vi "PickAndPlace.vi"(0 "Operations":T1={"GoToToolPos"=TRUE, "PickTool"=TRUE, "GoToSenPCB"=TRUE, "PickSiPCB"=TRUE, "GoToBP"=TRUE, "DropTool"=TRUE}, 1 "VacuumStates":path=path "C:/Users/TTUHEP/Documents/LabVIEW/GantryPrograms/Configs/PickPlaceVacuumStates.json", 2 "AssemblyPositions":path=path "C:/Users/TTUHEP/Documents/LabVIEW/GantryPrograms/Configs/BaseplatePositions.txt", 5 "AssmbType":enum16{"Sensor", "PCB"}(ring)=enum."PCB", 7 "Zone":enum16{"ZoneA", "ZoneB", "ZoneC", "ZoneD"}(ring), 9 "Position":enum16{"1", "2"}(ring), 11 "Error In":errorcluster, 12 "PUT_Positions":path=path "C:/Users/TTUHEP/Documents/LabVIEW/GantryPrograms/Configs/PUT_Positions.txt", 13 "SiPositions":path=path "C:/Users/TTUHEP/Documents/LabVIEW/GantryPrograms/Configs/SensorPositions.txt", 14 "PCBPositions":path=path "C:/Users/TTUHEP/Documents/LabVIEW/GantryPrograms/Configs/PCBPositions.txt") -> (4 "Log":string, 15 "Error Out":errorcluster)   [LabVIEW 2019]
panel:
  out "Assembly_XYZU":dbl[](array[numeric])
  out "PUT_XYZU":dbl[](array[numeric])
  out "PUT rotation":dbl
  in  "FastZDrop":dbl=65.0
  in  "FastZToolPick":dbl=85.0
  in  "FastZSiPCBPick":dbl=65.0
  in  "LineNo":u8
  in  "ZSpeed":dbl=10.0
  in  "XYSpeed":dbl=100.0
  out "SiPCBXYZU":dbl[](array[numeric])
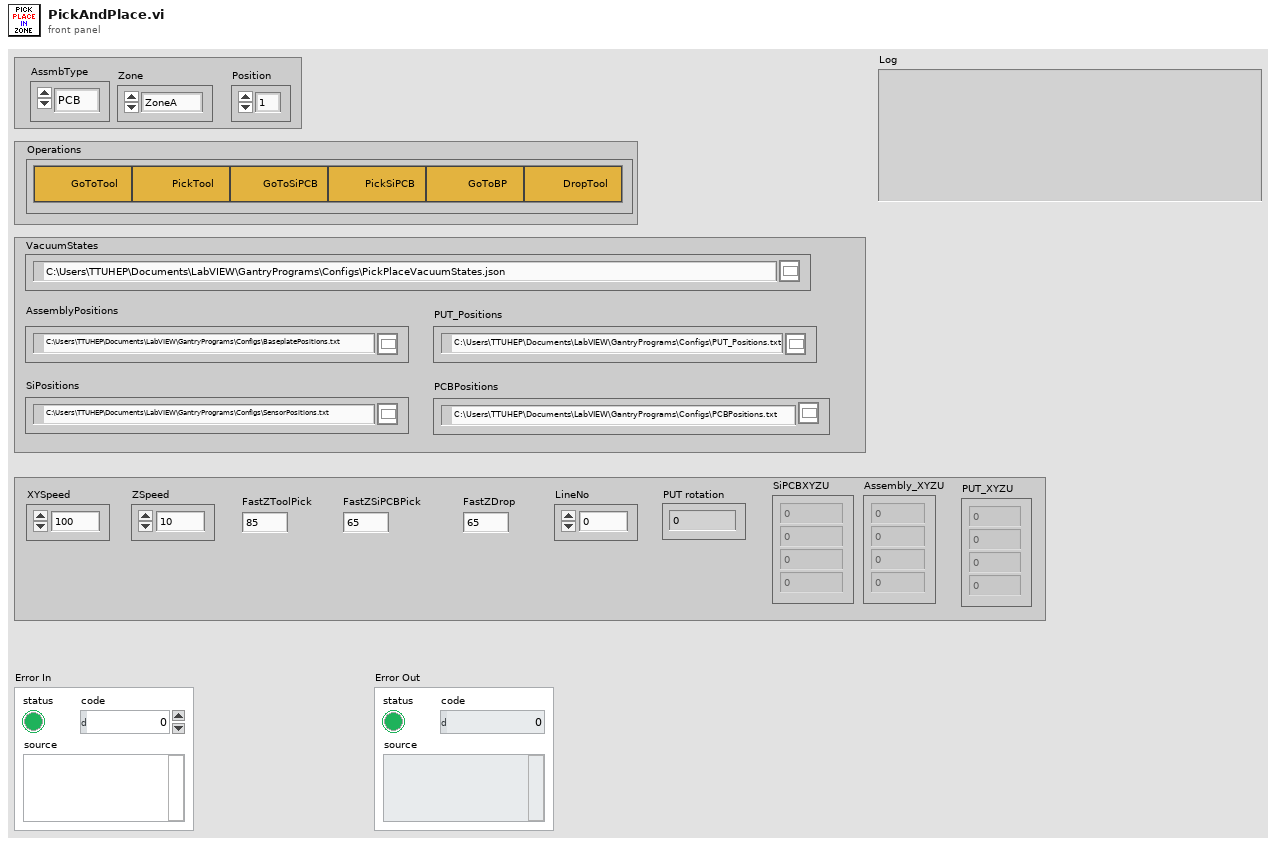
[diagram p1: front panel]
types:
  T1 = cluster{"GoToToolPos":bool, "PickTool":bool, "GoToSenPCB":bool, "PickSiPCB":bool, "GoToBP":bool, "DropTool":bool}
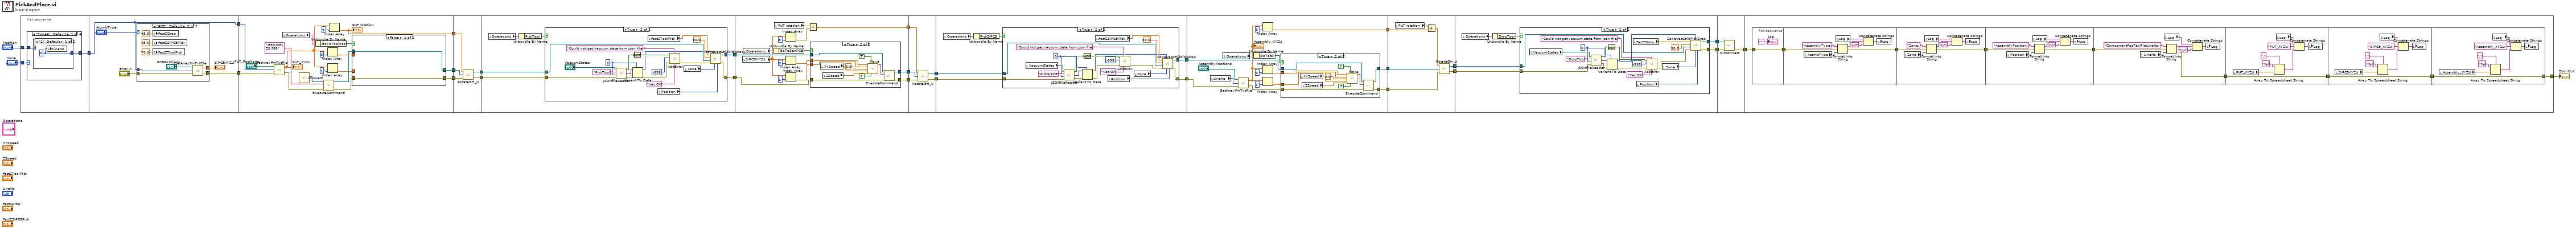
[diagram p0: block diagram]
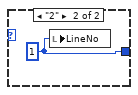
[diagram p2: hidden frame]
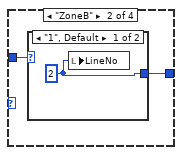
[diagram p3: hidden frame]
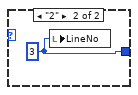
[diagram p4: hidden frame]
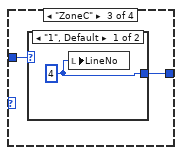
[diagram p5: hidden frame]
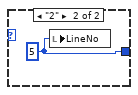
[diagram p6: hidden frame]
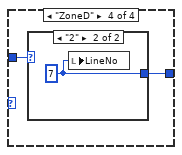
[diagram p7: hidden frame]
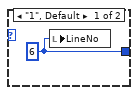
[diagram p8: hidden frame]
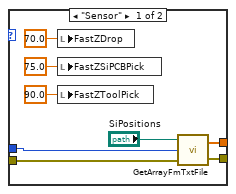
[diagram p9: hidden frame]
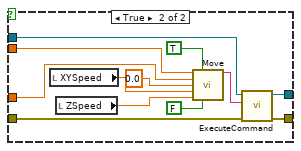
[diagram p10: hidden frame]
diagram:
  n1 = flat-sequence {
    tunnel: [w29] -> w8
    tunnel: "Zone" -> [w31]
    tunnel: "Position" -> [w30]
    tunnel: [w50] -> w9
    tunnel: w8 -> [w48]
    tunnel: [w48] -> w6
    tunnel: [w77] -> w28
    tunnel: [w76] -> w27
    tunnel: [w75] -> w26
    tunnel: w9 -> [w71]
    tunnel: w6 -> [w74]
    tunnel: w28 -> [w106]
    tunnel: w27 -> [w105]
    tunnel: w26 -> [w104]
    tunnel: [w103] -> w25
    tunnel: [w102] -> w24
    tunnel: w25 -> [w110]
    tunnel: w24 -> [w109]
    tunnel: [w108] -> w23
    tunnel: [w107] -> w22
    tunnel: w23 -> [w143]
    tunnel: w22 -> [w142]
    tunnel: [w136] -> w21
    tunnel: [w141] -> w20
    tunnel: [w140] -> w19
    tunnel: w21 -> [w169]
    tunnel: w20 -> [w168]
    tunnel: w19 -> [w167]
    tunnel: [w166] -> w18
    tunnel: [w165] -> w17
    tunnel: w18 -> [w173]
    tunnel: w17 -> [w172]
    tunnel: [w171] -> w16
    tunnel: [w170] -> w15
    tunnel: w16 -> [w205]
    tunnel: w15 -> [w204]
    tunnel: [w202] -> w14
    tunnel: [w201] -> w13
    tunnel: [w200] -> w12
    tunnel: w14 -> [w235]
    tunnel: w13 -> [w234]
    tunnel: w12 -> [w232]
    tunnel: [w230] -> w11
    tunnel: [w229] -> w10
    tunnel: w11 -> [w239]
    tunnel: w10 -> [w238]
    tunnel: [w237] -> w4
    tunnel: [w236] -> w3
    tunnel: w4 -> [w267]
    tunnel: w3 -> [w266]
    tunnel: [w265] -> w1
    tunnel: [w270] -> w2
    tunnel: w1 -> [w268]
    frame #0 {
      n2 = case shown="\"ZoneA\", Default" w31 {
        tunnel: w30 -> [w33 w37 w41 w45]
        tunnel: [w32 w36 w40 w44] -> w29
        frame "ZoneA", Default {
          n3 = case shown="\"1\", Default" w33 {
            tunnel: [w34 w35] -> w32
            frame "1", Default {
              w34 = u8 0 ("LineNo")
              n4 = local write "LineNo"(w34) -> ()
            }
            frame "2" {
              w35 = u8 1 ("LineNo")
              n5 = local write "LineNo"(w35) -> ()
            }
          }
        }
        frame "ZoneB" {
          n6 = case shown="\"1\", Default" w37 {
            tunnel: [w38 w39] -> w36
            frame "1", Default {
              w38 = u8 2 ("LineNo")
              n7 = local write "LineNo"(w38) -> ()
            }
            frame "2" {
              w39 = u8 3 ("LineNo")
              n8 = local write "LineNo"(w39) -> ()
            }
          }
        }
        frame "ZoneC" {
          n9 = case shown="\"1\", Default" w41 {
            tunnel: [w42 w43] -> w40
            frame "1", Default {
              w42 = u8 4 ("LineNo")
              n10 = local write "LineNo"(w42) -> ()
            }
            frame "2" {
              w43 = u8 5 ("LineNo")
              n11 = local write "LineNo"(w43) -> ()
            }
          }
        }
        frame "ZoneD" {
          n12 = case shown="\"2\"" w45 {
            tunnel: [w46 w47] -> w44
            frame "1", Default {
              w46 = u8 6 ("LineNo")
              n13 = local write "LineNo"(w46) -> ()
            }
            frame "2" {
              w47 = u8 7 ("LineNo")
              n14 = local write "LineNo"(w47) -> ()
            }
          }
        }
      }
    }
    frame #1 {
      n15 = case shown="\"PCB\", Default" "AssmbType" {
        tunnel: w48 -> [w59 w67]
        tunnel: [w58 w66] -> w52
        tunnel: "Error In" -> [w57 w65]
        tunnel: [w56 w64] -> w50
        frame "Sensor" {
          n16 = local write "FastZDrop"(70.0 ("FastZDrop")) -> ()
          n17 = local write "FastZSiPCBPick"(75.0 ("FastZSiPCBPick")) -> ()
          n18 = local write "FastZToolPick"(90.0 ("FastZToolPick")) -> ()
          n19 = call "GetArrayFmTxtFile.vi"("error in"=w57, "LineNo."=w59, "TextFile"="SiPositions") -> ("error out"=w56:errorcluster, "Array"=w58:dbl[])
        }
        frame "PCB", Default {
          n20 = local write "FastZDrop"(45.0 ("FastZDrop")) -> ()
          n21 = local write "FastZSiPCBPick"(45.0 ("FastZSiPCBPick")) -> ()
          n22 = local write "FastZToolPick"(70.0 ("FastZToolPick")) -> ()
          n23 = call "GetArrayFmTxtFile.vi"("error in"=w65, "LineNo."=w67, "TextFile"="PCBPositions") -> ("error out"=w64:errorcluster, "Array"=w66:dbl[])
        }
      }
      "SiPCBXYZU" <- w52
    }
    frame #2 {
      n24 = call "GetArrayFmTxtFile.vi"("error in"=w71, "LineNo."=w74, "TextFile"="PUT_Positions") -> ("error out"=w72:errorcluster, "Array"=w69:dbl[])
      "PUT_XYZU" <- w69
      n25 = local read "Operations"() -> (w84:T1)
      n26 = call "Connect.vi"() -> ("controller"=w70:refnum<k24>)  [unwired: 10 in, 1 out]
      n27 = Unbundle By Name(w84) -> ("GoToToolPos"=w83:bool)
      n28 = call "ExecuteCommand.vi"("error in (no error)"=w72, "Command Code"="G90\nG1 Z0 F50", "controller in"=w70) -> ("error out"=w87:errorcluster, "controller out"=w86:refnum<k24>)  [unwired: 6 in, 1 out]
      n29 = Index Array(array=w69, index=0) -> (element=w79:dbl)
      n30 = Index Array(array=w69, index=1) -> (element=w78:dbl)
      n31 = Index Array(array=w69, index=3) -> (element=w75:dbl)
      "PUT rotation" <- w75
      n32 = case shown="False" w83 {
        tunnel: w86 -> [w89 w98]
        tunnel: w87 -> [w88 w97]
        tunnel: [w88 w96] -> w77
        tunnel: [w89 w95] -> w76
        tunnel: w79 -> [_ w94]
        tunnel: w78 -> [_ w93]
        frame False {
        }
        frame True {
          n33 = local read "XYSpeed"() -> (w91:dbl)
          n34 = local read "ZSpeed"() -> (w90:dbl)
          n35 = call "Move.vi"("X"=w94, "Absolute"=TRUE, "Y"=w93, "Z"=0.0, "SpeedXY (mm/s)"=w91, "SpeedZ (mm/s)"=w90, "Move Z first"=FALSE) -> ("Position Gcode"=w99:string)  [unwired: 8 in]
          n36 = call "ExecuteCommand.vi"("error in (no error)"=w97, "Command Code"=w99, "controller in"=w98) -> ("error out"=w96:errorcluster, "controller out"=w95:refnum<k24>)  [unwired: 6 in, 1 out]
        }
      }
    }
    frame #3 {
      n37 = call "RotateGH_U.vi"("error in (no error)"=w106, "controller in"=w105, "U"=w104) -> ("error out"=w103:errorcluster, "controller out"=w102:refnum<k24>)
    }
    frame #4 {
      n38 = local read "Operations"() -> (w112:T1)
      n39 = Unbundle By Name(w112) -> ("PickTool"=w111:bool)
      n40 = case shown="True" w111 {
        tunnel: w110 -> [w114 w121]
        tunnel: w109 -> [w113 w134]
        tunnel: [w114 w117] -> w108
        tunnel: [w113 w116] -> w107
        frame False {
        }
        frame True {
          w124 = u8 0
          n41 = call "JSONfileReader.vi"("error in"=w121, "Variant"=w124, "ItemName"="PickTool", "FileIn"="VacuumStates") -> ("error out"=w119:errorcluster, "Data"=w123:variant, "Found"=w128:bool)
          n42 = Not(x=w128) -> (.not. x?=w129:bool)
          n43 = Variant To Data(error in=w119, type=w124, Variant=w123) -> (data=w122:u8, error out=w118:errorcluster)
          n44 = local read "FastZToolPick"() -> (w115:dbl)
          n45 = local read "Position"() -> (w133:enum16{"1", "2"})
          n46 = call "AddError.vi"("NoErrorMessage"="Vac OK", "ErrorMessage"="Could not get vacuum state from json file.", "error in"=w118, "code"=-998, "Error?"=w129) -> ("Error out"=w120:errorcluster)  [unwired: 6 in]
          n47 = local read "Zone"() -> (w132:enum16{"ZoneA", "ZoneB", "ZoneC", "ZoneD"})
          n48 = call "ZoneVacCtrldPickDrop.vi"("Position"=w133, "Zone"=w132, "VacuumState"=w122, "error in (no error)"=w120, "controller in"=w134, "Zspeed"=50.0, "Z"=w115) -> ("error out"=w117:errorcluster, "controller out"=w116:refnum<k24>)  [unwired: 3 in]
        }
      }
    }
    frame #5 {
      n49 = local read "SiPCBXYZU"() -> (w139:dbl[])
      n50 = local read "Operations"() -> (w147:T1)
      n51 = Unbundle By Name(w147) -> ("GoToSenPCB"=w148:bool)
      n52 = local read "PUT rotation"() -> (w138:dbl)
      n53 = Index Array(array=w139, index=3) -> (element=w137:dbl)
      n54 = Index Array(array=w139, index=0) -> (element=w149:dbl)
      n55 = Index Array(array=w139, index=1) -> (element=w150:dbl)
      n56 = Add(x=w138, y=w137) -> (x+y=w136:dbl)
      n57 = case shown="True" w148 {
        tunnel: w142 -> [w152 w161]
        tunnel: w143 -> [w151 w160]
        tunnel: [w151 w159] -> w140
        tunnel: [w152 w158] -> w141
        tunnel: w149 -> [_ w157]
        tunnel: w150 -> [_ w156]
        frame False {
        }
        frame True {
          n58 = local read "XYSpeed"() -> (w153:dbl)
          n59 = local read "ZSpeed"() -> (w154:dbl)
          n60 = call "Move.vi"("X"=w157, "Absolute"=TRUE, "Y"=w156, "Z"=0.0, "SpeedXY (mm/s)"=w153, "SpeedZ (mm/s)"=w154, "Move Z first"=FALSE) -> ("Position Gcode"=w162:string)  [unwired: 8 in]
          n61 = call "ExecuteCommand.vi"("error in (no error)"=w160, "Command Code"=w162, "controller in"=w161) -> ("error out"=w159:errorcluster, "controller out"=w158:refnum<k24>)  [unwired: 6 in, 1 out]
        }
      }
    }
    frame #6 {
      n62 = call "RotateGH_U.vi"("error in (no error)"=w167, "controller in"=w168, "U"=w169) -> ("error out"=w165:errorcluster, "controller out"=w166:refnum<k24>)
    }
    frame #7 {
      n63 = local read "Operations"() -> (w174:T1)
      n64 = Unbundle By Name(w174) -> ("PickSiPCB"=w175:bool)
      n65 = case shown="True" w175 {
        tunnel: w172 -> [w177 w186]
        tunnel: w173 -> [w176 w178]
        tunnel: [w177 w182] -> w170
        tunnel: [w176 w181] -> w171
        frame False {
        }
        frame True {
          w189 = u8 0
          n66 = local read "VacuumStates"() -> (w180:path)
          n67 = call "JSONfileReader.vi"("error in"=w186, "Variant"=w189, "ItemName"="PickSiPCB", "FileIn"=w180) -> ("error out"=w184:errorcluster, "Data"=w188:variant, "Found"=w193:bool)
          n68 = Not(x=w193) -> (.not. x?=w194:bool)
          n69 = Variant To Data(error in=w184, type=w189, Variant=w188) -> (data=w187:u8, error out=w183:errorcluster)
          n70 = local read "FastZSiPCBPick"() -> (w179:dbl)
          n71 = local read "Position"() -> (w197:enum16{"1", "2"})
          n72 = call "AddError.vi"("NoErrorMessage"="Vac OK", "ErrorMessage"="Could not get vacuum state from json file.", "error in"=w183, "code"=-998, "Error?"=w194) -> ("Error out"=w185:errorcluster)  [unwired: 6 in]
          n73 = local read "Zone"() -> (w196:enum16{"ZoneA", "ZoneB", "ZoneC", "ZoneD"})
          n74 = call "ZoneVacCtrldPickDrop.vi"("Position"=w197, "Zone"=w196, "VacuumState"=w187, "error in (no error)"=w185, "controller in"=w178, "Zspeed"=50.0, "Z"=w179) -> ("error out"=w182:errorcluster, "controller out"=w181:refnum<k24>)  [unwired: 3 in]
        }
      }
    }
    frame #8 {
      n75 = local read "LineNo"() -> (w206:u8)
      n76 = local read "Operations"() -> (w214:T1)
      n77 = call "GetArrayFmTxtFile.vi"("error in"=w204, "LineNo."=w206, "TextFile"="AssemblyPositions") -> ("error out"=w203:errorcluster, "Array"=w199:dbl[])
      "Assembly_XYZU" <- w199
      n78 = Unbundle By Name(w214) -> ("GoToBP"=w213:bool)
      n79 = Index Array(array=w199, index=3) -> (element=w200:dbl)
      n80 = Index Array(array=w199, index=0) -> (element=w212:dbl)
      n81 = Index Array(array=w199, index=1) -> (element=w211:dbl)
      n82 = case shown="True" w213 {
        tunnel: w205 -> [w216 w225]
        tunnel: w203 -> [w215 w224]
        tunnel: [w215 w223] -> w202
        tunnel: [w216 w222] -> w201
        tunnel: w212 -> [_ w221]
        tunnel: w211 -> [_ w220]
        frame False {
        }
        frame True {
          n83 = local read "XYSpeed"() -> (w217:dbl)
          n84 = local read "ZSpeed"() -> (w218:dbl)
          n85 = call "Move.vi"("X"=w221, "Absolute"=TRUE, "Y"=w220, "Z"=0.0, "SpeedXY (mm/s)"=w217, "SpeedZ (mm/s)"=w218, "Move Z first"=FALSE) -> ("Position Gcode"=w226:string)  [unwired: 8 in]
          n86 = call "ExecuteCommand.vi"("error in (no error)"=w224, "Command Code"=w226, "controller in"=w225) -> ("error out"=w223:errorcluster, "controller out"=w222:refnum<k24>)  [unwired: 6 in, 1 out]
        }
      }
    }
    frame #9 {
      n87 = local read "PUT rotation"() -> (w233:dbl)
      n88 = Add(x=w233, y=w232) -> (x+y=w231:dbl)
      n89 = call "RotateGH_U.vi"("error in (no error)"=w235, "controller in"=w234, "U"=w231) -> ("error out"=w230:errorcluster, "controller out"=w229:refnum<k24>)
    }
    frame #10 {
      n90 = local read "Operations"() -> (w241:T1)
      n91 = Unbundle By Name(w241) -> ("DropTool"=w240:bool)
      n92 = case shown="True" w240 {
        tunnel: w239 -> [w243 w247]
        tunnel: w238 -> [w242 w246]
        tunnel: [w243 w245] -> w237
        tunnel: [w242 w244] -> w236
        frame False {
        }
        frame True {
          w253 = u8 0
          n93 = local read "VacuumStates"() -> (w263:path)
          n94 = call "JSONfileReader.vi"("error in"=w247, "Variant"=w253, "ItemName"="DropTool", "FileIn"=w263) -> ("error out"=w261:errorcluster, "Data"=w258:variant, "Found"=w257:bool)
          n95 = Not(x=w257) -> (.not. x?=w256:bool)
          n96 = Variant To Data(error in=w261, type=w253, Variant=w258) -> (data=w259:u8, error out=w262:errorcluster)
          n97 = local read "FastZDrop"() -> (w264:dbl)
          n98 = local read "Position"() -> (w254:enum16{"1", "2"})
          n99 = call "AddError.vi"("NoErrorMessage"="Vac OK", "ErrorMessage"="Could not get vacuum state from json file.", "error in"=w262, "code"=-998, "Error?"=w256) -> ("Error out"=w260:errorcluster)  [unwired: 6 in]
          n100 = local read "Zone"() -> (w255:enum16{"ZoneA", "ZoneB", "ZoneC", "ZoneD"})
          n101 = call "ZoneVacCtrldPickDrop.vi"("Position"=w254, "Zone"=w255, "VacuumState"=w259, "error in (no error)"=w260, "controller in"=w246, "Zspeed"=50.0, "Z"=w264) -> ("error out"=w245:errorcluster, "controller out"=w244:refnum<k24>)  [unwired: 3 in]
        }
      }
    }
    frame #11 {
      n102 = call "Disconnect.vi"("error in (no error)"=w267, "controller"=w266) -> ("error out"=w265:errorcluster)  [unwired: 9 in]
    }
    frame #12 {
      n103 = flat-sequence {
        tunnel: [w277] -> w269
        tunnel: w268 -> [w277]
        tunnel: [w280] -> w276
        tunnel: w269 -> [w279]
        tunnel: w276 -> [w288]
        tunnel: [w287] -> w275
        tunnel: [w296] -> w274
        tunnel: w275 -> [w297]
        tunnel: w274 -> [w304]
        tunnel: [w303] -> w273
        tunnel: [w311] -> w272
        tunnel: w273 -> [w311]
        tunnel: [w319] -> w271
        tunnel: w272 -> [w319]
        tunnel: [w327] -> w270
        tunnel: w271 -> [w327]
        frame #0 {
          "Log" <- ""
        }
        frame #1 {
          n104 = local read "AssmbType"() -> (w286:enum16{"Sensor", "PCB"})
          n105 = local read "Log"() -> (w281:string)
          n106 = Format Into String(initial string="AssemblyType: ", error in=w279, w286) -> (resulting string=w283:string, error out=w280:errorcluster)  [unwired: 1 in]
          n107 = Concatenate Strings(w281, w283, "\r\n") -> (w285:string)
          n108 = local write "Log"(w285) -> ()
        }
        frame #2 {
          n109 = local read "Zone"() -> (w294:enum16{"ZoneA", "ZoneB", "ZoneC", "ZoneD"})
          n110 = local read "Log"() -> (w291:string)
          n111 = Format Into String(initial string="Zone: ", error in=w288, w294) -> (resulting string=w293:string, error out=w287:errorcluster)  [unwired: 1 in]
          n112 = Concatenate Strings(w291, w293, "\r\n") -> (w292:string)
          n113 = local write "Log"(w292) -> ()
        }
        frame #3 {
          n114 = local read "Position"() -> (w300:enum16{"1", "2"})
          n115 = local read "Log"() -> (w302:string)
          n116 = Format Into String(initial string="AssemblyPosition: ", error in=w297, w300) -> (resulting string=w301:string, error out=w296:errorcluster)  [unwired: 1 in]
          n117 = Concatenate Strings(w302, w301, "\r\n") -> (w295:string)
          n118 = local write "Log"(w295) -> ()
        }
        frame #4 {
          n119 = local read "LineNo"() -> (w310:u8)
          n120 = local read "Log"() -> (w308:string)
          n121 = Format Into String(initial string="ComponentPosTexFileLineNo: ", error in=w304, w310) -> (resulting string=w309:string, error out=w303:errorcluster)  [unwired: 1 in]
          n122 = Concatenate Strings(w308, w309, "\r\n") -> (w307:string)
          n123 = local write "Log"(w307) -> ()
        }
        frame #5 {
          n124 = local read "PUT_XYZU"() -> (w318:dbl[])
          n125 = Array To Spreadsheet String(delimiter (Tab)=",", array=w318, 3:"%f" ("format string")) -> (spreadsheet string=w315:string)
          n126 = local read "Log"() -> (w313:string)
          n127 = Concatenate Strings(w313, "PUT_XYZU: " ("string"), w315) -> (w314:string)
          n128 = local write "Log"(w314) -> ()
        }
        frame #6 {
          n129 = local read "SiPCBXYZU"() -> (w326:dbl[])
          n130 = Array To Spreadsheet String(delimiter (Tab)=",", array=w326, 3:"%f" ("format string")) -> (spreadsheet string=w323:string)
          n131 = local read "Log"() -> (w321:string)
          n132 = Concatenate Strings(w321, "SiPCB_XYZU: " ("string"), w323) -> (w322:string)
          n133 = local write "Log"(w322) -> ()
        }
        frame #7 {
          n134 = local read "Assembly_XYZU"() -> (w328:dbl[])
          n135 = Array To Spreadsheet String(delimiter (Tab)=",", array=w328, 3:"%f" ("format string")) -> (spreadsheet string=w333:string)
          n136 = local read "Log"() -> (w329:string)
          n137 = Concatenate Strings(w329, "Assembly_XYZU: " ("string"), w333) -> (w331:string)
          n138 = local write "Log"(w331) -> ()
        }
      }
    }
  }
  "Error Out" <- w2
